vi "data update.vi"(0 "tdms in":refnum<k34>, 1 "sample counter in":i32, 5 "cache in":T1, 7 "data table in":T2, 9 "Time Stamp":timestamp, 11 "error in":errorcluster, 12 "output type order":T3[](array[typedef]), 13 "scans per write":i32) -> (3 "sample counter out":i32, 4 "tdms out":refnum<k34>, 6 "cache out":T1, 8 "data table out":T2, 15 "error out":errorcluster)   [LabVIEW 2013, in "TDMS datalogger runtime.lvclass"]
uses:
  TDMS datalogger runtime.lvclass
  <vilib>/NI/Tag Bus/tag/Data Type.ctl
  data cache.ctl
  <vilib>/NI/Tag Bus/table/data table.ctl
  <vilib>/NI/Tag Bus/tag/tag descriptor.lvclass
  <vilib>/NI/Tag Bus/table/data table.lvlib
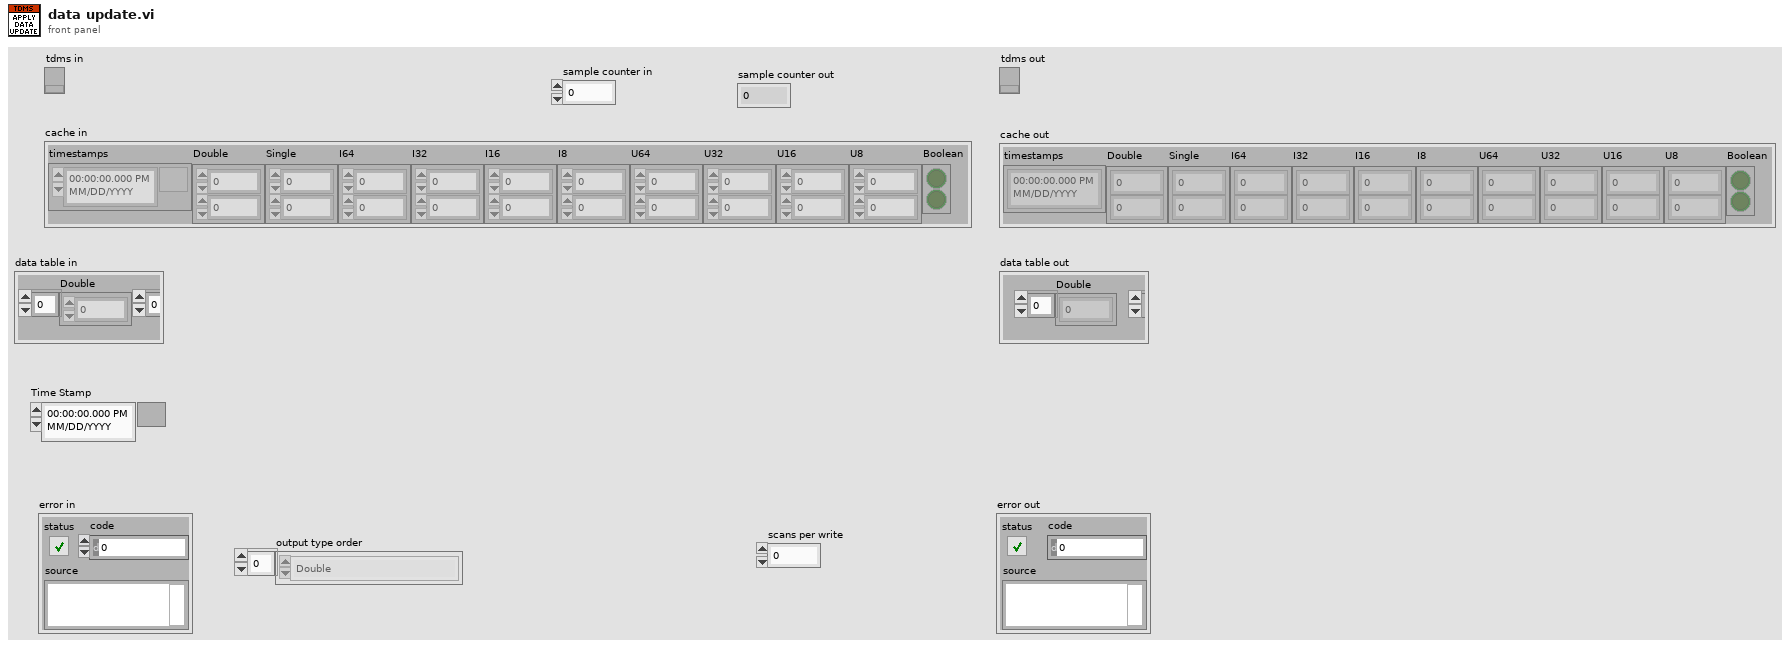
[diagram p1: front panel]
types:
  T1 = typedef "TDMS datalogger runtime.lvclass/data cache.ctl" = cluster{"timestamps":timestamp[], "Double":dbl[][], "Single":sgl[][], "I64":i64[][], "I32":i32[][], "I16":i16[][], "I8":i8[][], "U64":u64[][], "U32":u32[][], "U16":u16[][], "U8":u8[][], "Boolean":bool[][]}
  T2 = typedef "tag bus.lvlib/data table.lvlib/data table.ctl" = cluster{"Double":dbl[], "Single":sgl[], "I64":i64[], "I32":i32[], "I16":i16[], "I8":i8[], "U64":u64[], "U32":u32[], "U16":u16[], "U8":u8[], "Boolean":bool[], "String":string[], "Array of Double":cluster{"DBL Array":dbl[]}[], "Array of Single":cluster{"SGL Array":sgl[]}[], "Array of I64":cluster{"I64 Array":i64[]}[], "Array of I32":cluster{"I32 Array":i32[]}[], "Array of I16":cluster{"I16 Array":i16[]}[], "Array of I8":cluster{"I8 Array":i8[]}[], "Array of U64":cluster{"U64 Array":u64[]}[], "Array of U32":cluster{"U32 Array":u32[]}[], "Array of U16":cluster{"U16 Array":u16[]}[], "Array of U8":cluster{"U8 Array":u8[]}[], "Array of Boolean":cluster{"Boolean Array":bool[]}[], "Array of String":cluster{"String Array":string[]}[]}
  T3 = typedef "tag bus.lvlib/tag descriptor.lvclass/Data Type.ctl" = enum16{"Double", "Single", "I64", "I32", "I16", "I8", "U64", "U32", "U16", "U8", "Boolean", "String", "Array of Double", "Array of Single", "Array of I64", "Array of I32", "Array of I16", "Array of I8", "Array of U64", "Array of U32", "Array of U16", "Array of U8", "Array of Boolean", "Array of String"}
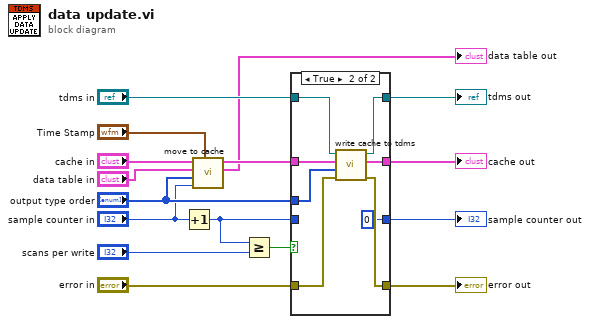
[diagram p0: block diagram]
diagram:
  n1 = Increment(x="sample counter in") -> (x+1=w16:i32)
  n2 = call "move to cache.vi"("Time Stamp"="Time Stamp", "sample counter"="sample counter in", "output type order"="output type order", "data table in"="data table in", "cache in"="cache in") -> ("data table out"=→"data table out":T2, "cache out"=w8:T1)  [unwired: 5 in]
  n3 = Greater Or Equal?(x=w16, y="scans per write") -> (x >= y?=w7:bool)
  n4 = case shown="True" w7 {
    tunnel: w8 -> [w20 w28]
    tunnel: [w20 w25] -> w9
    tunnel: "output type order" -> [_ w26]
    tunnel: "error in" -> [w18 w27]
    tunnel: [w18 w24] -> w12
    tunnel: [w19 w23] -> w13
    tunnel: "tdms in" -> [w19 w22]
    tunnel: [w17 0] -> w15
    tunnel: w16 -> [w17 _]
    frame False {
    }
    frame True {
      n5 = call "write cache to tdms.vi"("error in"=w27, "output type order"=w26, "cache in"=w28, "tdms file in"=w22) -> ("error out"=w24:errorcluster, "cache out"=w25:T1, "tdms file out"=w23:refnum<k34>)  [unwired: 5 in]
    }
  }
  "sample counter out" <- w15
  "tdms out" <- w13
  "error out" <- w12
  "cache out" <- w9
